vi "Write RHS.lvclass.vi"(8 "error in (no error)":errorcluster, 10 "RHS.lvclass":refnum<class "NI_RHS.lvclass">, 11 "PDE.lvclass in":refnum<class "NI_PDE.lvclass">) -> (0 "error out":errorcluster, 3 "PDE.lvclass out":refnum<class "NI_PDE.lvclass">)   [LabVIEW 2017, in "NI_PDE.lvlib" / "NI_PDE.lvclass"]
uses:
  <vilib>/gmath/pde.llb/PDEClass/NI_PDE.lvclass
  <vilib>/gmath/pde.llb/RHSClass/NI_RHS.lvclass
  <vilib>/gmath/pde.llb/PDEClass/NI_PDE.lvclass/NI_PDE.ctl
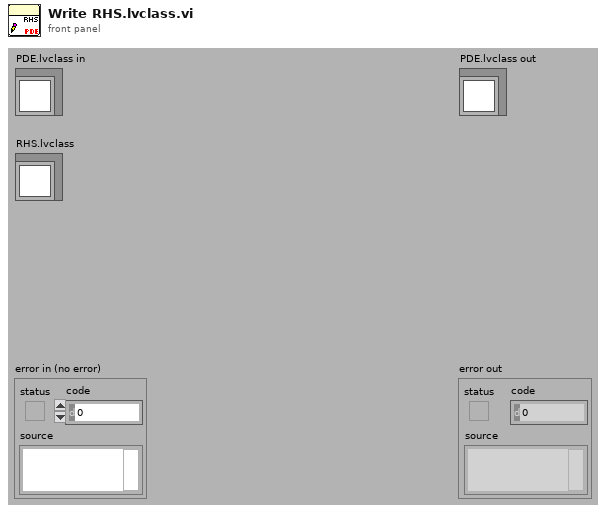
[diagram p1: front panel]
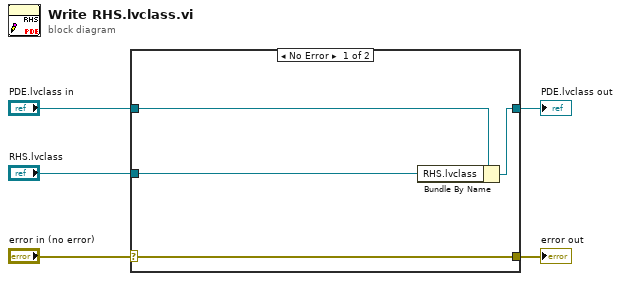
[diagram p0: block diagram]
diagram:
  n1 = case shown="No Error" "error in (no error)" {
    selector: "error in (no error)" -> [w9 w10]
    tunnel: [w9 w10] -> w4
    tunnel: [w7 w11] -> w2
    tunnel: "PDE.lvclass in" -> [w8 w11]
    tunnel: "RHS.lvclass" -> [w6 _]
    frame No Error {
      n2 = Bundle By Name(cluster=w8, "RHS.lvclass"=w6) -> (w7:refnum<class "NI_PDE.lvclass">)
    }
    frame Error {
    }
  }
  "error out" <- w4
  "PDE.lvclass out" <- w2
